vi "processSubVIs.vi"(7 "VIDependencyPaths":path[](array[path]), 8 "error in (no error)":errorcluster, 9 "SubVIs[]":refnum<vi>[](array[refnum]), 10 "Calling VI Reference i":refnum<vi>, 11 "Dependency in":refnum<class "Dependency.lvclass">) -> (0 "error out":errorcluster, 2 "Calling VI Reference o":refnum<vi>, 3 "Dependency out":refnum<class "Dependency.lvclass">)   [LabVIEW 2016, in "Dependency.lvclass"]
uses:
  Dependency.lvclass
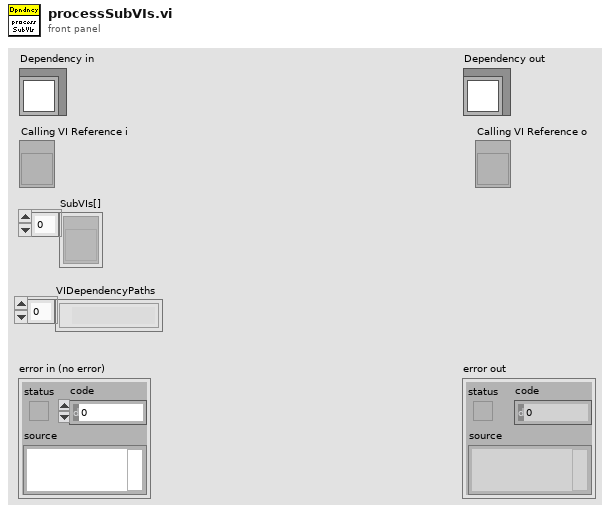
[diagram p1: front panel]
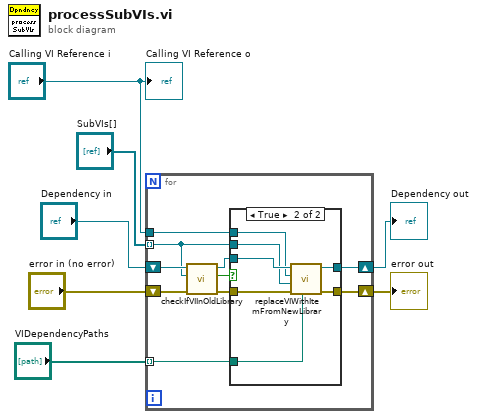
[diagram p0: block diagram]
diagram:
  n1 = for {
    shift-right: [w15] -> w2
    shift-left: "Dependency in" -> [w17]
    tunnel: "SubVIs[]" -> [w12] mode=indexing
    tunnel: "Calling VI Reference i" -> [w13]
    tunnel: "VIDependencyPaths" -> [w11] mode=indexing
    shift-right: [w8] -> w6
    shift-left: "error in (no error)" -> [w10]
    n2 = call "checkIfVIInOldLibrary.vi"("error in (no error)"=w10, "element"=w12, "Dependency in"=w17) -> ("error out"=w9:errorcluster, "isMemberOfOldLibrary"=w14:bool, "Dependency out"=w16:refnum<class "Dependency.lvclass">)  [unwired: 5 in, 1 out]
    n3 = case shown="True" w14 {
      tunnel: w16 -> [w19 w26]
      tunnel: [w19 w25] -> w15
      tunnel: w13 -> [_ w24]
      tunnel: w12 -> [_ w23]
      tunnel: w11 -> [_ w20]
      tunnel: w9 -> [w18 w22]
      tunnel: [w18 w21] -> w8
      frame False {
      }
      frame True {
        n4 = call "replaceVIWithItemFromNewLibrary.vi"("SubVI Path"=w20, "error in (no error)"=w22, "SubVI Refnum"=w23, "Calling VI Reference"=w24, "Dependency in"=w26) -> ("error out"=w21:errorcluster, "Dependency out"=w25:refnum<class "Dependency.lvclass">)  [unwired: 5 in]
      }
    }
  }
  "error out" <- w6
  "Dependency out" <- w2
  "Calling VI Reference o" <- "Calling VI Reference i"
